vi "Parse using dll.vi"() -> ()   [LabVIEW 2015]
uses:
  D:/Metis Automation/ppt-parsing/CSharp/ParsePpt/ParsePpt/bin/Debug/ParsePpt.dll
  CSharp/ParsePpt/ParsePpt/bin/Debug/ParsePpt.dll
panel:
  in  "Path":path
  out "ImageParts":string[](array[string])
  out "TextParts":string[](array[string])
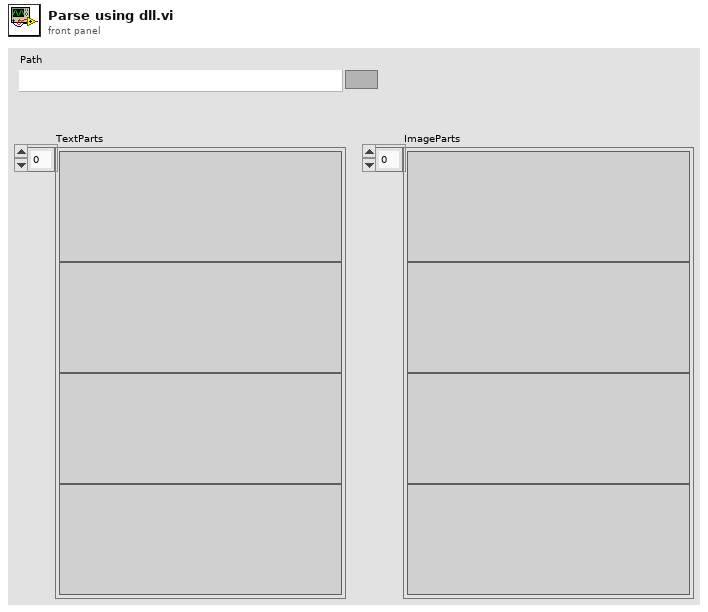
[diagram p1: front panel]
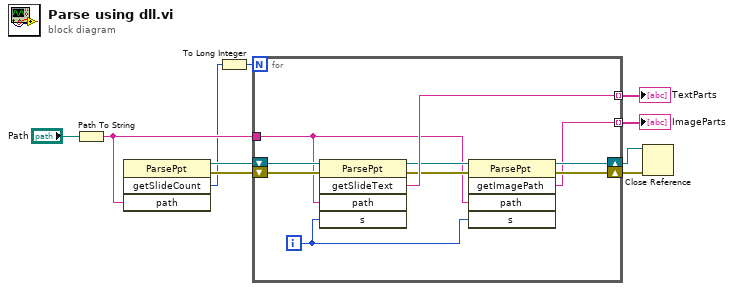
[diagram p0: block diagram]
diagram:
  n1 = Path To String(path="Path") -> (string=w6:string)
  n2 = invoke class="ParsePpt" method="getSlideCount"("path"=w6) -> (reference out=w8:refnum<k24>, error out=w7:errorcluster, "getSlideCount"=w4:i64)  [unwired: 3 in, 1 out]
  n3 = To Long Integer(number=w4) -> (32bit integer=w3:i32)
  n4 = for {
    N: w3 -> [_]
    shift-right: [w16] -> w9
    shift-left: w8 -> [w20]
    shift-right: [w14] -> w10
    shift-left: w7 -> [w19]
    tunnel: w6 -> [w12]
    tunnel: [w18] -> w5 mode=indexing
    tunnel: [w11] -> w2 mode=indexing
    i -> [w13]
    n5 = invoke class="ParsePpt" method="getSlideText"(reference=w20, error in=w19, "path"=w12, "s"=w13) -> (reference out=w17:refnum<k24>, error out=w15:errorcluster, "getSlideText"=w18:string)  [unwired: 1 in, 2 out]
    n6 = invoke class="ParsePpt" method="getImagePath"(reference=w17, error in=w15, "path"=w12, "s"=w13) -> (reference out=w16:refnum<k24>, error out=w14:errorcluster, "getImagePath"=w11:string)  [unwired: 1 in, 2 out]
  }
  "TextParts" <- w5
  "ImageParts" <- w2
  n7 = Close Reference(reference=w9, error in (no error)=w10) -> ()  [unwired: 1 out]
